vi "send_instruction.vi"(8 "error in":errorcluster, 9 "IP Address":string, 10 "Parameters":u8[](array[numeric]), 11 "Instruction":u8) -> (0 "error out":errorcluster, 2 "Return Values":u8[](array[numeric]))   [LabVIEW 2014]
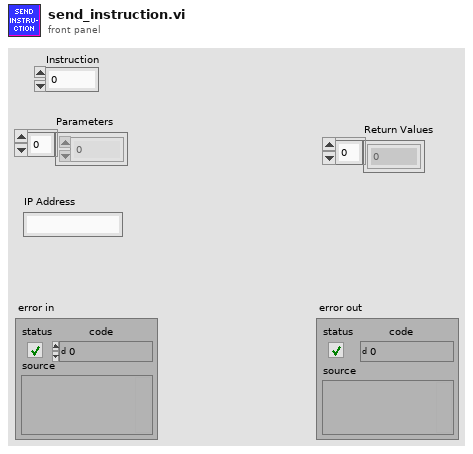
[diagram p1: front panel]
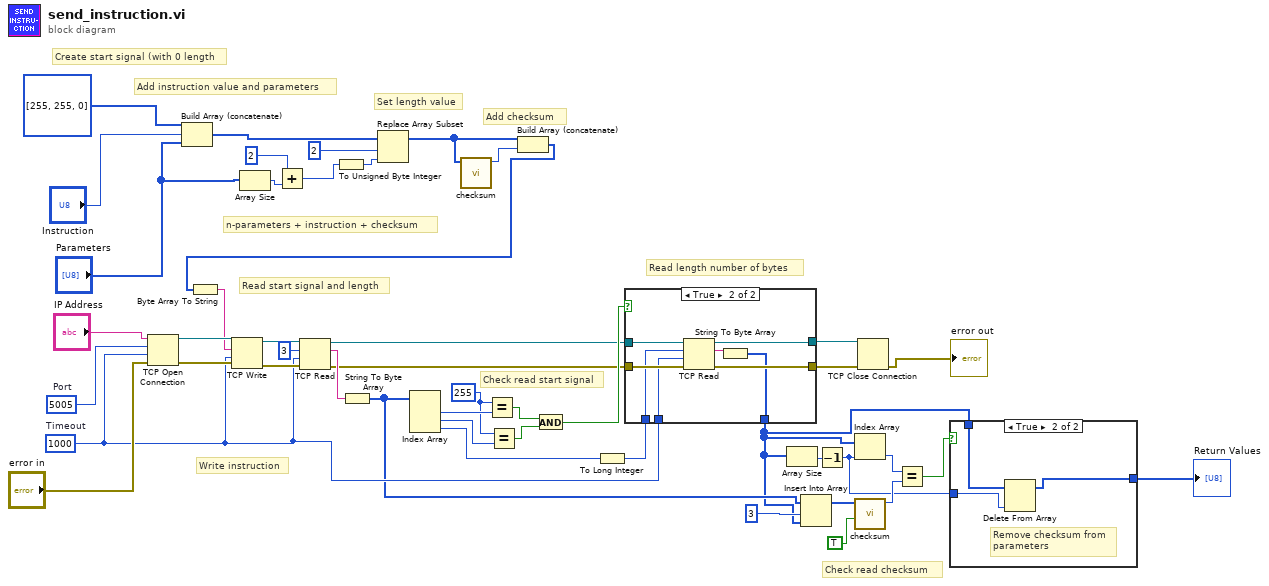
[diagram p0: block diagram]
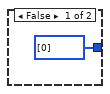
[diagram p2: hidden frame]
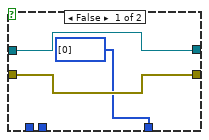
[diagram p3: hidden frame]
diagram:
  w25 = u8 255 ("x")
  w45 = u16 5005  # Port
  w17 = 1000  # Timeout
  # "Read length number of bytes"
  # "Check read checksum"
  # "Check read start signal"
  # "Read start signal and length"
  # "Write instruction"
  # "Add checksum"
  # "n-parameters + instruction + checksum"
  # "Set length value"
  # "Add instruction value and parameters"
  # "Create start signal (with 0 length"
  n1 = TCP Open Connection(address="IP Address", remote port or service name=w45, timeout ms (60000)=w17, error in (no error)="error in") -> (connection ID=w43:refnum<k5>, error out=w44:errorcluster)  [unwired: 1 in]
  n2 = Build Array (concatenate)(u8[] [255, 255, 0], "Instruction", "Parameters") -> (w39:u8[])
  n3 = Array Size(array="Parameters") -> (size(s)=w40:i32)
  n4 = Add(x=2, y=w40) -> (x+y=w36:i32)
  n5 = To Unsigned Byte Integer(number=w36) -> (unsigned 8bit integer=w37:u8)
  n6 = Replace Array Subset(array=w39, new element=w37, index=2) -> (w35:u8[])
  n7 = call "checksum.vi"("Array"=w35) -> ("unsigned 8bit integer"=w34:u8)  [unwired: 10 in]
  n8 = Build Array (concatenate)(w35, w34) -> (w33:u8[])
  n9 = Byte Array To String(unsigned byte array=w33) -> (string=w32:string)
  n10 = TCP Write(connection ID=w43, data in=w32, error in (no error)=w44, 9:w17) -> (connection ID out=w31:refnum<k5>, error out=w30:errorcluster)  [unwired: 1 out]
  n11 = TCP Read(connection ID=w31, bytes to read=3, error in (no error)=w30, 9:w17) -> (connection ID out=w21:refnum<k5>, data out=w28:string, error out=w20:errorcluster)  [unwired: 1 in]
  n12 = String To Byte Array(string=w28) -> (unsigned byte array=w14:u8[])
  n13 = Index Array(array=w14) -> (element #1=w27:u8, element #2=w26:u8, element #3=w19:u8)  [unwired: 3 in]
  n14 = Equal?(x=w25, y=w27) -> (x = y?=w24:bool)
  n15 = Equal?(x=w25, y=w26) -> (x = y?=w23:bool)
  n16 = And(x=w24, y=w23) -> (x .and. y?=w22:bool)
  n17 = To Long Integer(number=w19) -> (32bit integer=w18:i32)
  n18 = case shown="True" w22 {
    tunnel: w21 -> [w50 w57]
    tunnel: w20 -> [w49 w58]
    tunnel: w18 -> [_ w56]
    tunnel: w17 -> [_ w55]
    tunnel: [w50 w54] -> w15
    tunnel: [w49 w53] -> w16
    tunnel: [u8[] [0] w51] -> w6
    frame False {
    }
    frame True {
      n19 = TCP Read(connection ID=w57, bytes to read=w56, error in (no error)=w58, 9:w55) -> (connection ID out=w54:refnum<k5>, data out=w52:string, error out=w53:errorcluster)  [unwired: 1 in]
      n20 = String To Byte Array(string=w52) -> (unsigned byte array=w51:u8[])
    }
  }
  n21 = Array Size(array=w6) -> (size(s)=w10:i32)
  n22 = Insert Into Array(array=w14, index=3, new element=w6) -> (w13:u8[])
  n23 = Decrement(x=w10) -> (x-1=w5:i32)
  n24 = Index Array(array=w6, index=w5) -> (element=w9:u8)
  n25 = call "checksum.vi"("Ignore last term"=TRUE, "Array"=w13) -> ("unsigned 8bit integer"=w11:u8)  [unwired: 9 in]
  n26 = TCP Close Connection(connection ID=w15, error in (no error)=w16) -> (error out=→"error out":errorcluster)  [unwired: 1 in, 1 out]
  n27 = Equal?(x=w9, y=w11) -> (x = y?=w7:bool)
  n28 = case shown="True" w7 {
    tunnel: w6 -> [_ w62]
    tunnel: w5 -> [_ w61]
    tunnel: [u8[] [0] ("unsigned byte array") w60] -> w4
    frame False {
    }
    frame True {
      # "Remove checksum from parameters"
      n29 = Delete From Array(array=w62, index=w61) -> (array with subset deleted=w60:u8[])  [unwired: 1 in, 1 out]
    }
  }
  "Return Values" <- w4
